vi "Write.vi"(8 "Error In":errorcluster, 10 "Data":u8[](array[numeric]), 11 "Channel In":refnum<class "Channel.lvclass">) -> (0 "Error Out":errorcluster, 2 "Write Count":u64, 3 "Channel Out":refnum<class "Channel.lvclass">)   [LabVIEW 2021, in "Field_RnD_Services_LIBSSH2_Toolkit.lvlib" / "Channel.lvclass"]
doc: "Writes binary data to the SSH channel represented by this Channel object. Only the first 30KB of the binary data will be written to the remote SSH server because of a hard-coded 30KB maximum data length in the libssh2 shared library. For binary data greater than 30KB, the <B>Write All</B> VI should be used instead."
uses:
  Channel.lvclass
  Channel.lvclass/Channel.ctl
  Session/Session.lvclass
  Field_RnD_Services_LIBSSH2_Toolkit.lvlib
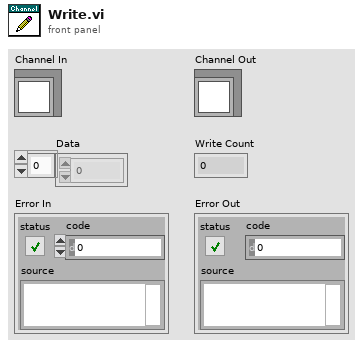
[diagram p1: front panel]
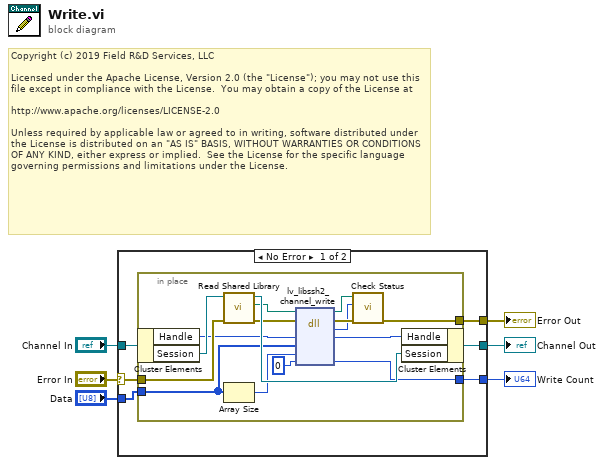
[diagram p0: block diagram]
diagram:
  # "Copyright (c) 2019 Field R&D Services, LLC\n\nLicensed under the Apache License, Version 2.0 (the \"License\"); you may not use this file except in compliance with the License.  You may obtain a copy of the License at\n\nhttp://www.apache.org/licenses/LICENSE-2.0\n\nUnless required by applicable law or agreed to in writing, software distributed under the License is distributed on an \"AS IS\" BASIS, WITHOUT WARRANTIES OR CONDITIONS OF ANY KIND, either express or implied.  See the License for the specific language governing permissions and limitations under the License."
  n1 = case shown="No Error" "Error In" {
    selector: "Error In" -> [w10 w29]
    tunnel: [w9 w29] -> w5
    tunnel: "Channel In" -> [w12 w28]
    tunnel: [w11 w28] -> w3
    tunnel: "Data" -> [w8 _]
    tunnel: [w7 _] -> w1
    frame No Error {
      n2 = in-place {
        in-place-border: w10 -> [w23]
        in-place-border: [w19] -> w9
        in-place-border: w8 -> [w15]
        in-place-border: [w13] -> w7
        n3 = in-place-cluster #1(w12) -> ("Handle"=w18:u64, "Session"=w27:refnum<class "Session.lvclass">)
        n4 = call "Read Shared Library.vi"("Error In"=w23, "Session In"=w27) -> ("Erorr Out"=w24:errorcluster, "libssh2lv Shared Library"=w25:path, "Session Out"=w26:refnum<class "Session.lvclass">)  [unwired: 7 in]
        n5 = Array Size(array=w15) -> (size(s)=w14:i32)
        n6 = dll-call lib="?" fn="lv_libssh2_channel_write"(path in=w25, error in=w24, "handle"=w18, "buffer"=w15, "buffer_len"=w14, "byte_count"=u64 0) -> (path out=w21:path, error out=w22:errorcluster, "status"=w20:i32, "handle"=w17:u64, "byte_count"=w13:u64)  [unwired: 3 in]
        n7 = call "Check Status.vi"("Error In"=w22, "Status"=w20, "libssh2lv Shared Library In"=w21) -> ("Error Out"=w19:errorcluster)  [unwired: 7 in, 1 out]
        n8 = in-place-cluster #1("Handle"=w17, "Session"=w26) -> (w11:refnum<class "Channel.lvclass">)
      }
    }
    frame Error {
    }
  }
  "Error Out" <- w5
  "Channel Out" <- w3
  "Write Count" <- w1
